vi "DCCM Analyze DC Current Measurements.vi"(0 "Current Waveforms":waveform(dbl)[](array[waveform]), 11 "error in (no error)":errorcluster) -> (4 "DC and RMS Current Measurements":T1 {"RMS Current (A)" format="%#.2p"; "Average DC Current (A)" format="%#.2p"}, 15 "error out":errorcluster)   [LabVIEW 2021, in "DAQ_DC-RMS Current Measurement.lvlib"]
doc: "Analyzes the DC current waveform data to derive required DC-RMS current measurements"
uses:
  DAQ_DC-RMS Current Measurement.lvlib
  Typedefs/DC and RMS Current Measurements.ctl
  <vilib>/measure/madcrms.llb/Basic Averaged DC-RMS for N Chan.vi
  <vilib>/measure/NI_MAPro.lvlib
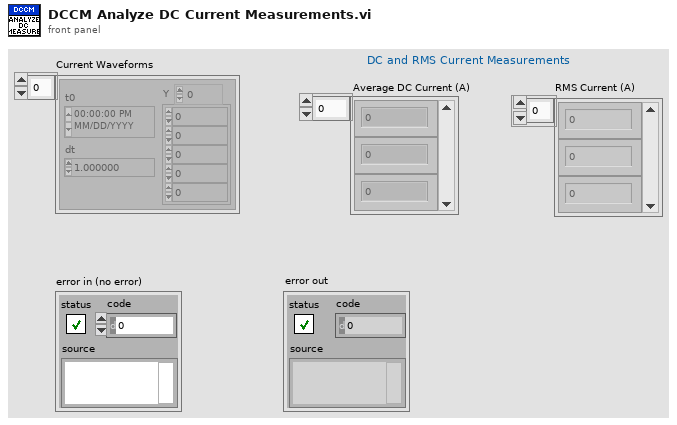
[diagram p1: front panel]
types:
  T1 = typedef "DAQ_DC-RMS Current Measurement.lvlib/DC and RMS Current Measurements.ctl" = cluster{"Average DC Current (A)":dbl[], "RMS Current (A)":dbl[]}
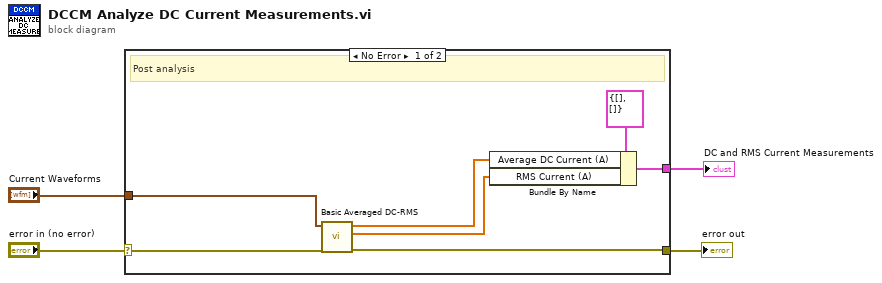
[diagram p0: block diagram]
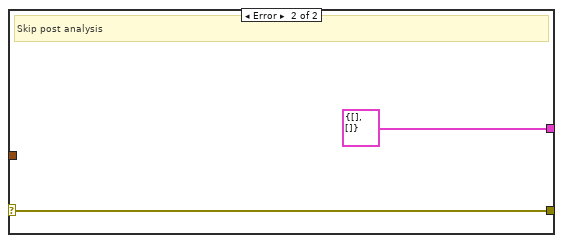
[diagram p2: hidden frame]
diagram:
  n1 = case shown="No Error" "error in (no error)" {
    selector: "error in (no error)" -> [w11 w12]
    tunnel: "Current Waveforms" -> [w10 _]
    tunnel: [w6 T1 {"Average DC Current (A)"=[], "RMS Current (A)"=[]} ("DC Measurements")] -> w1
    tunnel: [w5 w12] -> w2
    frame No Error {
      # "Post analysis"
      n2 = call-poly <vilib>:"Basic Averaged DC-RMS.vi"("error in (no error)"=w11, "signals in"=w10) -> ("error out"=w5:errorcluster, "RMS values"=w7:dbl[], "DC values"=w8:dbl[])  [unwired: 6 in, 1 out]
      n3 = Bundle By Name(cluster=T1 {"Average DC Current (A)"=[], "RMS Current (A)"=[]} ("DC Measurements"), "Average DC Current (A)"=w8, "RMS Current (A)"=w7) -> (w6:T1)
    }
    frame Error {
      # "Skip post analysis"
    }
  }
  "error out" <- w2
  "DC and RMS Current Measurements" <- w1
